vi "ReversedEngineering CreateOneStateNode.vi"(0 "Add Actions":bool, 1 "State":string, 2 "Actions":string[](array[string]), 3 "Comments":string[](array[string]), 5 "error in":errorcluster, 6 "Add Comments":bool, 7 "GraphRefToAddNodesTo":refnum<class "Graph.lvclass">, 9 "graphics":refnum<class "Graphics.lvclass">, 11 "grid":refnum<class "Grid.lvclass">) -> (14 "reference out":refnum<class "AbstractNode.lvclass">, 15 "bounds":T1 {"height" format="%.2f"; "width" format="%.2f"; "y" format="%.2f"; "x" format="%.2f"}, 19 "error out":errorcluster)   [LabVIEW 2020]
uses:
  <resource>/Framework/Providers/Open_GDS/UML/AbstractNode_class/AbstractNode.lvclass
  <resource>/Framework/Providers/Open_GDS/UML/Grid_class/Grid.lvclass
  <resource>/Framework/Providers/Open_GDS/UML/Graphics_class/Graphics.lvclass
  <resource>/Framework/Providers/Open_GDS/UML/Graph_class/Graph.lvclass
  <resource>/Framework/Providers/Open_GDS/UML/General/Rectangle/Rectangle Rectangle2D.ctl
  <resource>/Framework/Providers/Open_GDS/UML/InitialStateNode_class/InitialStateNode.lvclass
  C:/Program Files (x86)/National Instruments/LabVIEW 2020/resource/Framework/Providers/Open_GDS/UML/RectangularNode_class/RectangularNode.lvclass
  <resource>/Framework/Providers/Open_GDS/UML/FinalStateNode_class/FinalStateNode.lvclass
  <resource>/Framework/Providers/Open_GDS/UML/StateNode_class/StateNode.lvclass
  <resource>/Framework/Providers/Open_GDS/UML/RectangularNode_class/RectangularNode.lvclass
  C:/Program Files (x86)/National Instruments/LabVIEW 2020/resource/Framework/Providers/Open_GDS/UML/AbstractNode_class/AbstractNode.lvclass
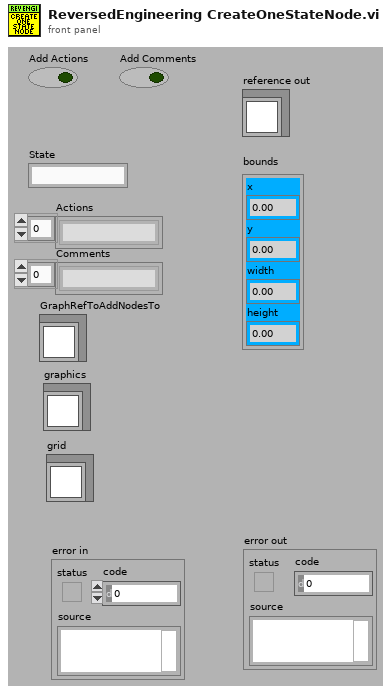
[diagram p1: front panel]
types:
  T1 = typedef "Rectangle Rectangle2D.ctl" = cluster{"x":dbl, "y":dbl, "width":dbl, "height":dbl}
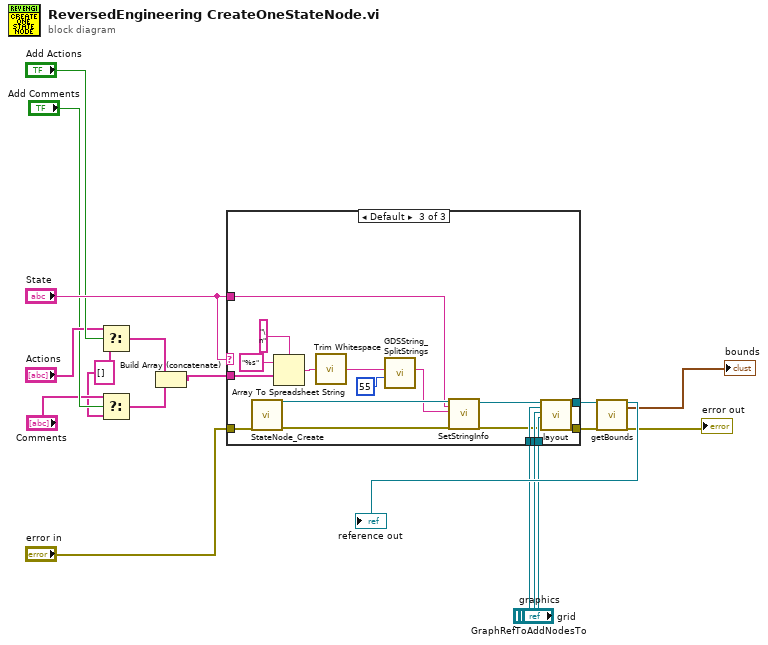
[diagram p0: block diagram]
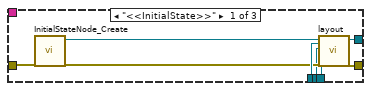
[diagram p2: hidden frame]
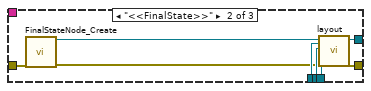
[diagram p3: hidden frame]
diagram:
  w2 = string[] [] ("f")
  n1 = Select(t="Actions", s="Add Actions", f=w2) -> (s? t:f=w5:string[])
  n2 = Select(t="Comments", s="Add Comments", f=w2) -> (s? t:f=w1:string[])
  n3 = Build Array (concatenate)(w5, w1) -> (w8:string[])
  n4 = case shown="Default" "State" {
    tunnel: "GraphRefToAddNodesTo" -> [w25 w34 w52]
    tunnel: "graphics" -> [w20 w31 w51]
    tunnel: "grid" -> [w19 w30 w50]
    tunnel: [w23 w33 w49] -> w13
    tunnel: [w22 w32 w48] -> w14
    tunnel: "State" -> [_ _ w43]
    tunnel: "error in" -> [w26 w29 w42]
    tunnel: w8 -> [_ _ w41]
    frame "<<InitialState>>" {
      n5 = call <resource>:"InitialStateNode_Create.vi"("error in (no error)"=w26) -> ("reference out"=w24:refnum<class "InitialStateNode.lvclass">, "error out"=w21:errorcluster)  [unwired: 1 in, 16 out]
      n6 = call-dynamic "layout.vi"("reference"=w24, "graph"=w25, "graphics"=w20, "grid"=w19, "error in (no error)"=w21) -> ("reference out"=w23:refnum<class "InitialStateNode.lvclass">, "error out"=w22:errorcluster)  [unwired: 13 in]
    }
    frame "<<FinalState>>" {
      n7 = call <resource>:"FinalStateNode_Create.vi"("error in (no error)"=w29) -> ("reference out"=w27:refnum<class "FinalStateNode.lvclass">, "error out"=w28:errorcluster)  [unwired: 1 in, 16 out]
      n8 = call-dynamic "layout.vi"("reference"=w27, "graph"=w34, "graphics"=w31, "grid"=w30, "error in (no error)"=w28) -> ("reference out"=w33:refnum<class "FinalStateNode.lvclass">, "error out"=w32:errorcluster)  [unwired: 13 in]
    }
    frame Default {
      n9 = call <resource>:"StateNode_Create.vi"("error in (no error)"=w42) -> ("reference out"=w47:refnum<class "StateNode.lvclass">, "error out"=w46:errorcluster)  [unwired: 1 in, 16 out]
      n10 = Array To Spreadsheet String(delimiter (Tab)="\n", array=w41, 3:"%s" ("format string")) -> (spreadsheet string=w40:string)
      n11 = call <vilib>:"Trim Whitespace.vi"("string"=w40) -> ("trimmed string"=w37:string)  [unwired: 1 in]
      n12 = call <resource>:"GDSString_SplitStrings.vi"("MaxCharactersPerRow(25)"=55, "StringIn"=w37) -> ("String Out"=w36:string)  [unwired: 9 in]
      n13 = call <resource>:"SetStringInfo.vi"("reference"=w47, "State"=w43, "Action"=w36, "error in (no error)"=w46) -> ("reference out"=w44:refnum<class "StateNode.lvclass">, "error out"=w45:errorcluster)  [unwired: 14 out]
      n14 = call-dynamic "layout.vi"("reference"=w44, "graph"=w52, "graphics"=w51, "grid"=w50, "error in (no error)"=w45) -> ("reference out"=w49:refnum<class "StateNode.lvclass">, "error out"=w48:errorcluster)  [unwired: 13 in]
    }
  }
  n15 = call-dynamic "getBounds.vi"("reference"=w13, "error in (no error)"=w14) -> ("reference out"=→"reference out":refnum<class "RectangularNode.lvclass">, "bounds"=→"bounds":T1, "error out"=→"error out":errorcluster)  [unwired: 15 in]
